vi "LVClass_CorrectionDataManager SetMicrolensesFocalLength.vi"(0 "CorrectionDataManager in":refnum<class "CorrectionDataManager.lvclass">, 5 "MicrolensesFocalLength":sgl, 11 "error in (no error)":errorcluster) -> (4 "CorrectionDataManager out":refnum<class "CorrectionDataManager.lvclass">, 15 "error out":errorcluster)   [LabVIEW 2020, in "CorrectionDataManager.lvclass"]
doc: "Wavefront corrector actuators count getter.\n\n--------------------------------------------------------------------------------\n\n<B>corrdata_managerIn </B> : CorrDataManager object.\n<B>corrdata_managerOut </B> : CorrDataManager object.\n<B>actuators_count </B> : WavefrontCorrector actuators count.\n<B>ErrorIn </B> : Error\n<B>ErrorOut </B> : Error\n\n--------------------------------------------------------------------------------"
uses:
  CorrectionDataManager.lvclass
  CorrectionDataManager.lvclass/CorrectionDataManager.ctl
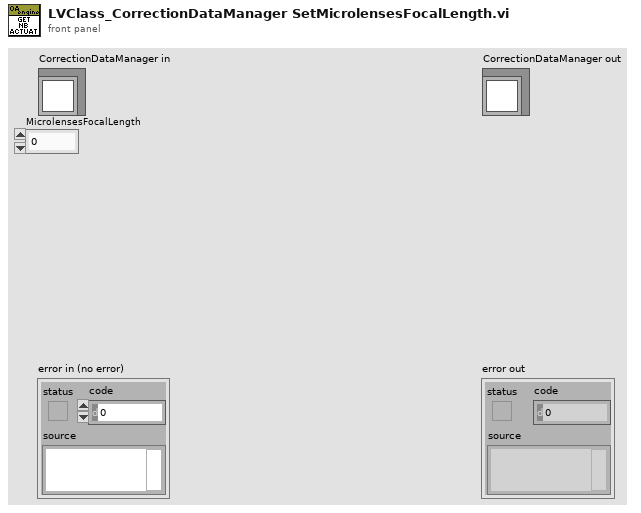
[diagram p1: front panel]
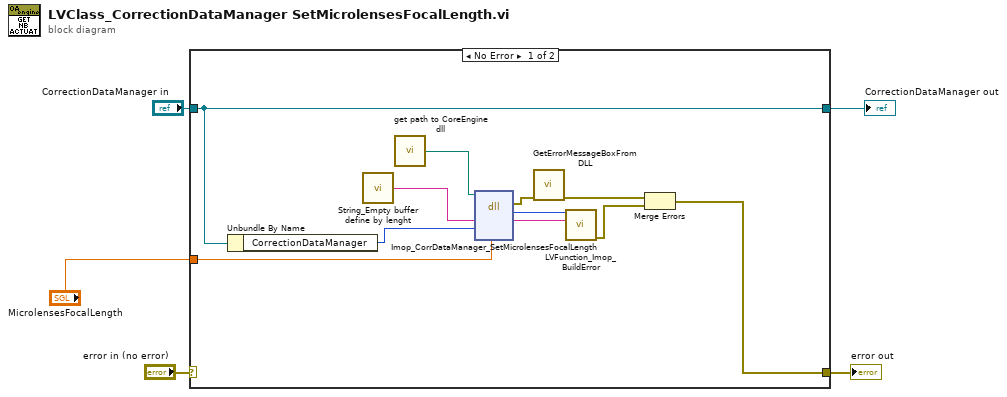
[diagram p0: block diagram]
diagram:
  n1 = case shown="No Error" "error in (no error)" {
    selector: "error in (no error)" -> [_ w18]
    tunnel: [w9 w18] -> w3
    tunnel: [w8 w17] -> w2
    tunnel: "CorrectionDataManager in" -> [w8 w17]
    tunnel: "MicrolensesFocalLength" -> [w6 _]
    frame No Error {
      n2 = Unbundle By Name(w8) -> ("CorrectionDataManager"=w7:i32)
      n3 = call "String_Empty buffer define by lenght.vi"() -> ("Empty buffer"=w14:string)  [unwired: 1 in]
      n4 = call "get path to CoreEngine dll.vi"() -> ("path to c_interface_vc100.dll"=w13:path)  [unwired: 12 in, 3 out]
      n5 = dll-call lib="D:/soft/HASO_v3/SVN_trunk/ImOpCoreEngine4_LV2011/DLLs/c_interface_vc100.dll" fn="Imop_CorrDataManager_SetMicrolensesFocalLength"(path in=w13, "message"=w14, "WavefrontCorrection"=w7, "MicrolensesFocalLength"=w6) -> (error out=w12:errorcluster, "return type"=w16:i32, "message"=w15:string)  [unwired: 4 in, 1 out]
      n6 = call "GetErrorMessageBoxFromDLL.vi"("error IN"=w12) -> ("error OUT"=w11:errorcluster)  [unwired: 10 in]
      n7 = call "LVFunction_Imop_BuildError.vi"("code"=w16, "String to Prepend to source (\"\")"=w15) -> ("error out"=w10:errorcluster)  [unwired: 13 in]
      n8 = Merge Errors(w11, w10) -> (w9:errorcluster)
    }
    frame Error {
    }
  }
  "error out" <- w3
  "CorrectionDataManager out" <- w2
